vi "Assert String Not Contains String.vi"(5 "Needle":string, 7 "Message (\"\")":string, 8 "error in (no error)":errorcluster, 10 "Haystack":string) -> (0 "error out":errorcluster)   [LabVIEW 2017, in "Transparent Assertions.lvlib"]
doc: "Asserts that a string does not contain the expected substring. Returns an error if the assertion fails, and optionally appends a custom message to the error."
uses:
  Transparent Assertions.lvlib
  LogicalNot/LogicalNot.lvclass
  StringContains/StringContains.lvclass
  C:/Users/pasca/Projects/Home/TransparentAssertions/src/Transparent Assertions/Constraints/Constraint/Constraint.lvclass
  UnaryOperator/UnaryOperator.lvclass
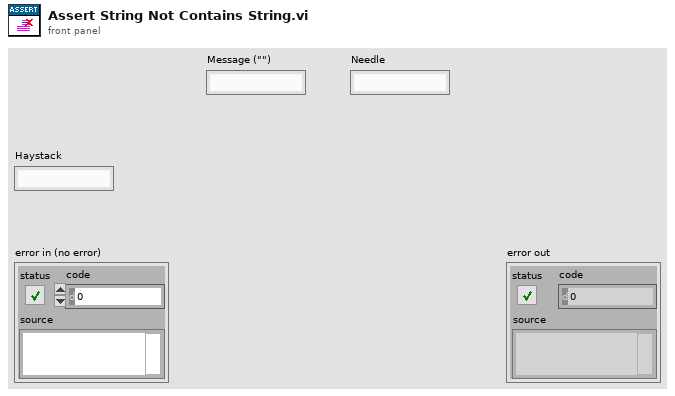
[diagram p1: front panel]
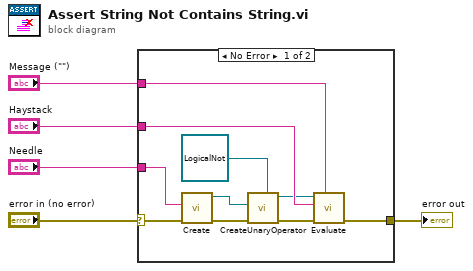
[diagram p0: block diagram]
diagram:
  n1 = case shown="No Error" "error in (no error)" {
    selector: "error in (no error)" -> [w11 w16]
    tunnel: "Haystack" -> [w14 _]
    tunnel: [w13 w16] -> w4
    tunnel: "Message (\"\")" -> [w12 _]
    tunnel: "Needle" -> [w10 _]
    frame No Error {
      n2 = call "Create.vi"("error in (no error)"=w11, "Needle"=w10) -> ("error out"=w15:errorcluster, "StringContains"=w7:refnum<class "StringContains.lvclass">)  [unwired: 8 in]
      n3 = call-dynamic "CreateUnaryOperator.vi"("UnaryOperator In"=refnum<class "LogicalNot.lvclass"> refnum ("Constraint.lvlib:LogicalNot.lvclass"), "error in (no error)"=w15, "Constraint"=w7) -> ("error out"=w9:errorcluster, "UnaryOperator"=w6:refnum<class "UnaryOperator.lvclass">)  [unwired: 7 in]
      n4 = call-dynamic "Evaluate.vi"("Message (\"\")"=w12, "error in (no error)"=w9, "Actual"=w14, "Constraint in"=w6) -> ("error out"=w13:errorcluster)  [unwired: 6 in, 1 out]
    }
    frame Error {
    }
  }
  "error out" <- w4
